vi "SetFrontPanelSize.vi"(4 "Top (-32768: unchange)":i16=-32768, 6 "Left (-32768: unchange)":i16=-32768, 7 "Relative (F)":bool, 8 "error in (no error)":errorcluster, 9 "Height (0: unchange)":i16, 10 "Width (0: unchange)":i16, 11 "VI Reference":refnum<vi>) -> (0 "error out":errorcluster, 3 "VI Reference out":refnum<vi>)   [LabVIEW 2021]
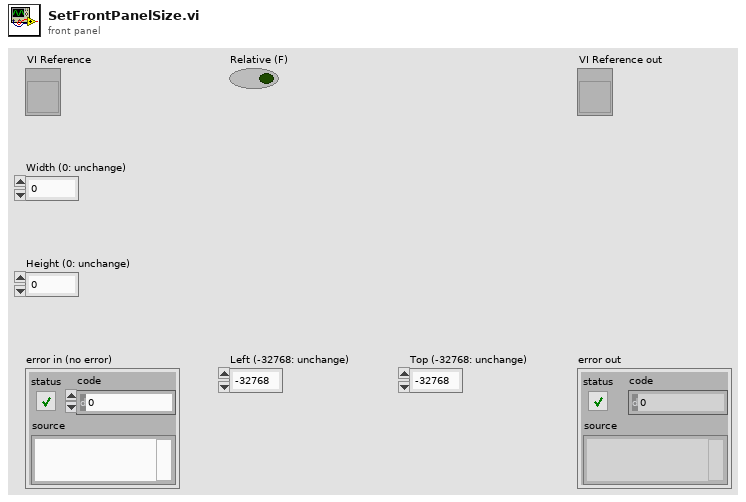
[diagram p1: front panel]
types:
  T1 = typedef "LVRectTypeDef.ctl" = cluster{"Left":i16, "Top":i16, "Right":i16, "Bottom":i16}
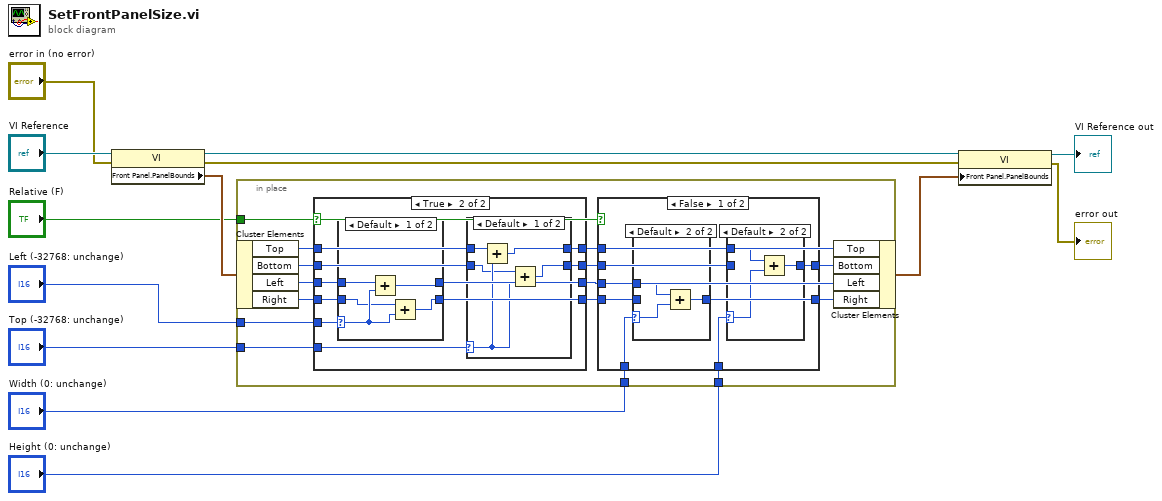
[diagram p0: block diagram]
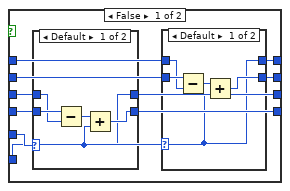
[diagram p2: hidden frame]
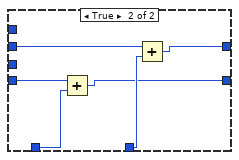
[diagram p9: hidden frame]
diagram:
  n1 = property class="VI"(reference="VI Reference", error in="error in (no error)") -> (reference out=w13:refnum<vi>, error out=w1:errorcluster, "Front Panel.PanelBounds"=w12:T1)
  n2 = in-place {
    in-place-border: "Width (0: unchange)" -> [w28]
    in-place-border: "Height (0: unchange)" -> [w27]
    in-place-border: "Relative (F)" -> [w24]
    in-place-border: "Left (-32768: unchange)" -> [w26]
    in-place-border: "Top (-32768: unchange)" -> [w25]
    n3 = in-place-cluster #1(w12) -> ("Top"=w23:i16, "Bottom"=w22:i16, "Left"=w21:i16, "Right"=w20:i16)
    n4 = case shown="True" w24 {
      tunnel: w26 -> [w38 w62]
      tunnel: [w37 w61] -> w14
      tunnel: [w36 w60] -> w19
      tunnel: w25 -> [w35 w59]
      tunnel: [w34 w58] -> w15
      tunnel: [w33 w57] -> w16
      tunnel: w23 -> [w29 w56]
      tunnel: w22 -> [w30 w55]
      tunnel: w21 -> [w31 w54]
      tunnel: w20 -> [w32 w53]
      frame False {
        n5 = case shown="Default" w38 {
          selector: w38 -> [w48 _]
          tunnel: [w48 w52] -> w37
          tunnel: [w50 w51] -> w36
          tunnel: w32 -> [w47 w51]
          tunnel: w31 -> [w46 w52]
          frame Default {
            n6 = Subtract(x=w47, y=w46) -> (x-y=w49:i16)
            n7 = Add(x=w49, y=w48) -> (x+y=w50:i16)
          }
          frame -32768 {
          }
        }
        n8 = case shown="Default" w35 {
          selector: w35 -> [w41 _]
          tunnel: [w41 w45] -> w34
          tunnel: [w42 w44] -> w33
          tunnel: w30 -> [w40 w44]
          tunnel: w29 -> [w39 w45]
          frame Default {
            n9 = Subtract(x=w40, y=w39) -> (x-y=w43:i16)
            n10 = Add(x=w43, y=w41) -> (x+y=w42:i16)
          }
          frame -32768 {
          }
        }
      }
      frame True {
        n11 = case shown="Default" w62 {
          selector: w62 -> [w72 _]
          tunnel: [w73 w76] -> w61
          tunnel: [w74 w75] -> w60
          tunnel: w54 -> [w71 w76]
          tunnel: w53 -> [w70 w75]
          frame Default {
            n12 = Add(x=w71, y=w72) -> (x+y=w73:i16)
            n13 = Add(x=w70, y=w72) -> (x+y=w74:i16)
          }
          frame -32768 {
          }
        }
        n14 = case shown="Default" w59 {
          selector: w59 -> [w66 _]
          tunnel: [w65 w69] -> w58
          tunnel: [w67 w68] -> w57
          tunnel: w56 -> [w64 w69]
          tunnel: w55 -> [w63 w68]
          frame Default {
            n15 = Add(x=w64, y=w66) -> (x+y=w65:i16)
            n16 = Add(x=w63, y=w66) -> (x+y=w67:i16)
          }
          frame -32768 {
          }
        }
      }
    }
    n17 = case shown="False" w24 {
      tunnel: w28 -> [w84 w97]
      tunnel: [w83 w96] -> w18
      tunnel: [w82 w95] -> w17
      tunnel: w27 -> [w81 w98]
      tunnel: w14 -> [w80 _]
      tunnel: w15 -> [w79 _]
      tunnel: w19 -> [w78 w94]
      tunnel: w16 -> [w77 w93]
      frame False {
        n18 = case shown="Default" w84 {
          selector: w84 -> [_ w87]
          tunnel: [w85 w88] -> w83
          tunnel: w80 -> [_ w86]
          tunnel: w78 -> [w85 _]
          frame 0 {
          }
          frame Default {
            n19 = Add(x=w86, y=w87) -> (x+y=w88:i16)
          }
        }
        n20 = case shown="Default" w81 {
          selector: w81 -> [_ w92]
          tunnel: [w89 w91] -> w82
          tunnel: w79 -> [_ w90]
          tunnel: w77 -> [w89 _]
          frame 0 {
          }
          frame Default {
            n21 = Add(x=w90, y=w92) -> (x+y=w91:i16)
          }
        }
      }
      frame True {
        n22 = Add(x=w94, y=w97) -> (x+y=w96:i16)
        n23 = Add(x=w93, y=w98) -> (x+y=w95:i16)
      }
    }
    n24 = in-place-cluster #1("Top"=w15, "Bottom"=w17, "Left"=w14, "Right"=w18) -> (w11:T1)
  }
  n25 = property class="VI"(reference=w13, error in=w1, "Front Panel.PanelBounds"=w11) -> (reference out=→"VI Reference out":refnum<vi>, error out=→"error out":errorcluster)
